vi "Calculate Voltage Pulses.vi"(0 "Stage Voltage Section":dbl[](array[numeric]), 5 "Stage.Dwell.Level":dbl, 7 "Active Edge":bool) -> (4 "# of Pulses":dbl)   [LabVIEW 2019, in "Fuel Injector Analysis Addon Engine.lvlib"]
uses:
  Fuel Injector Analysis Addon Engine.lvlib
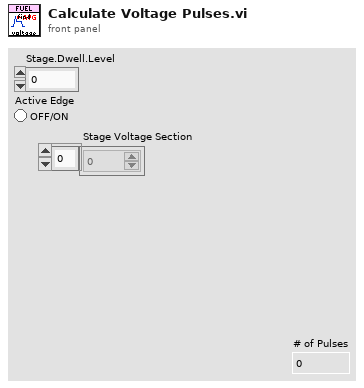
[diagram p1: front panel]
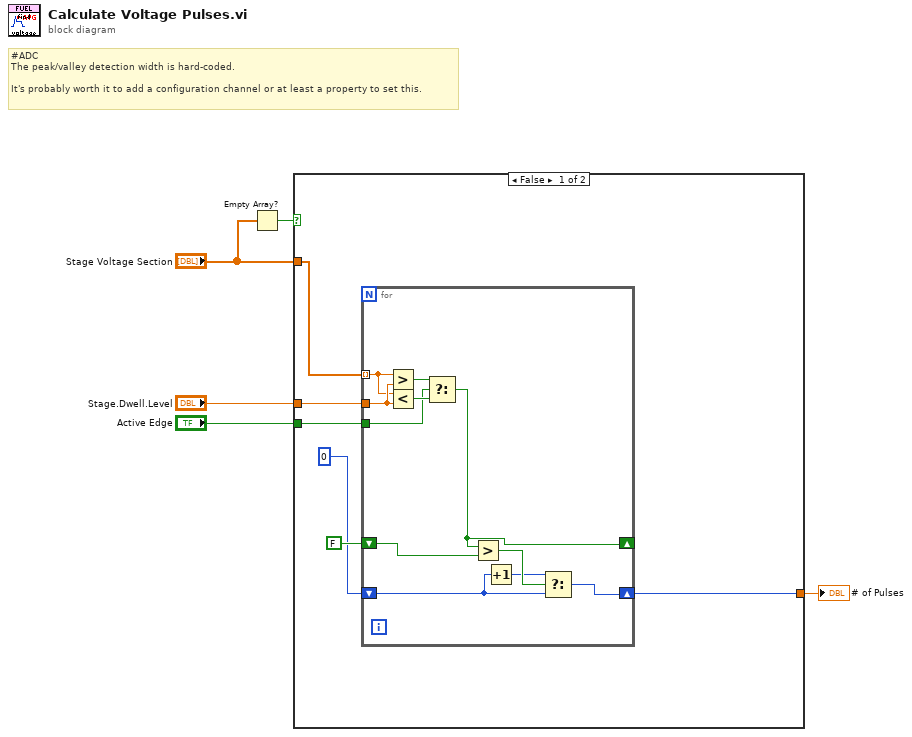
[diagram p0: block diagram]
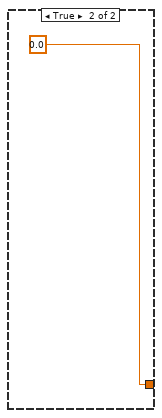
[diagram p2: hidden frame]
diagram:
  # "#ADC \nThe peak/valley detection width is hard-coded.\n\nIt's probably worth it to add a configuration channel or at least a property to set this."
  n1 = Empty Array?(array="Stage Voltage Section") -> (empty?=w2:bool)
  n2 = case shown="False" w2 {
    tunnel: [w9 0.0 ("mean")] -> w5
    tunnel: "Stage.Dwell.Level" -> [w8 _]
    tunnel: "Stage Voltage Section" -> [w7 _]
    tunnel: "Active Edge" -> [w6 _]
    frame False {
      n3 = for {
        tunnel: w7 -> [w16] mode=indexing
        tunnel: w8 -> [w17]
        shift-right: [w13] -> _
        shift-left: FALSE -> [w22]
        shift-right: [w20] -> w9
        shift-left: 0 -> [w19]
        tunnel: w6 -> [w12]
        n4 = Greater?(x=w16, y=w17) -> (0:w15:bool)
        n5 = Less?(x=w16, y=w17) -> (x < y?=w14:bool)
        n6 = Select(t=w15, s=w12, f=w14) -> (s? t:f=w13:bool)
        n7 = Greater?(x=w13, y=w22) -> (0:w21:bool)
        n8 = Increment(x=w19) -> (x+1=w18:i32)
        n9 = Select(t=w18, s=w21, f=w19) -> (s? t:f=w20:i32)
      }
    }
    frame True {
    }
  }
  "# of Pulses" <- w5
